vi "ReadData.vi"(8 "error in (no error)":errorcluster, 11 "DataBank in":refnum<class "DataBank.lvclass">) -> (0 "error out":errorcluster, 2 "Data":T1, 3 "DataBank out":refnum<class "DataBank.lvclass">)   [LabVIEW 2012, in "DataBank.lvclass"]
uses:
  DataBank.lvclass
  DataBank.lvclass/DataBank.ctl
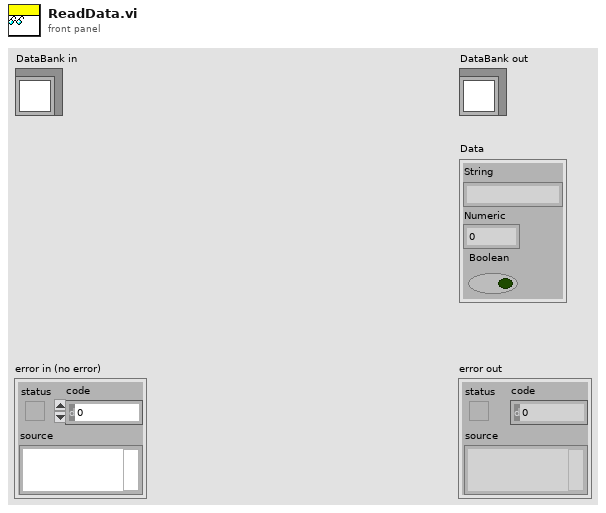
[diagram p1: front panel]
types:
  T1 = cluster{"String":string, "Numeric":i32, "Boolean":bool}
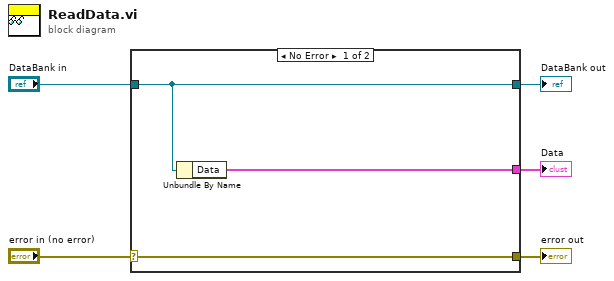
[diagram p0: block diagram]
diagram:
  n1 = case shown="No Error" "error in (no error)" {
    selector: "error in (no error)" -> [w8 w9]
    tunnel: [w8 w9] -> w4
    tunnel: [w7 w10] -> w2
    tunnel: "DataBank in" -> [w7 w10]
    tunnel: [w6 _] -> w1
    frame No Error {
      n2 = Unbundle By Name(w7) -> ("Data"=w6:T1)
    }
    frame Error {
    }
  }
  "error out" <- w4
  "DataBank out" <- w2
  "Data" <- w1
